vi "Min-Max Check.vi"(9 "Minimum":dbl, 10 "Maximum":dbl, 11 "Input":dbl) -> (3 "Output":dbl)   [LabVIEW 2015]
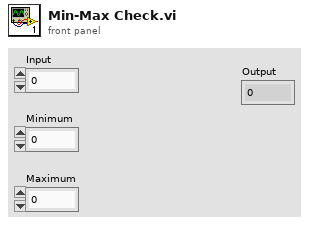
[diagram p1: front panel]
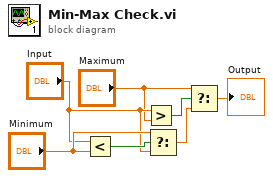
[diagram p0: block diagram]
diagram:
  n1 = Less?(x="Input", y="Minimum") -> (x < y?=w7:bool)
  n2 = Greater?(x="Input", y="Maximum") -> (0:w3:bool)
  n3 = Select(t="Minimum", s=w7, f="Input") -> (s? t:f=w5:dbl)
  n4 = Select(t="Maximum", s=w3, f=w5) -> (s? t:f=→"Output":dbl)
